vi "Read Controls.vi"(8 "error in (no error)":errorcluster, 11 "Test.Maui 2.0.Panels in":refnum<class "Test.Maui 2.0.Panels.lvclass">) -> (0 "error out":errorcluster, 2 "Controls":T1(array[cluster]), 3 "Test.Maui 2.0.Panels out":refnum<class "Test.Maui 2.0.Panels.lvclass">)   [LabVIEW 2020, in "Test.Maui 2.0.Panels.lvclass"]
uses:
  Test.Maui 2.0.Panels.lvclass
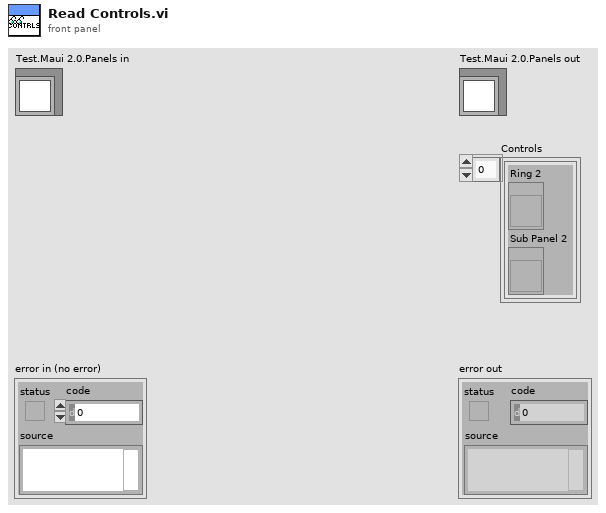
[diagram p1: front panel]
types:
  T1 = cluster{"Ring 2":refnum<vi>, "Sub Panel 2":refnum<vi>}[]
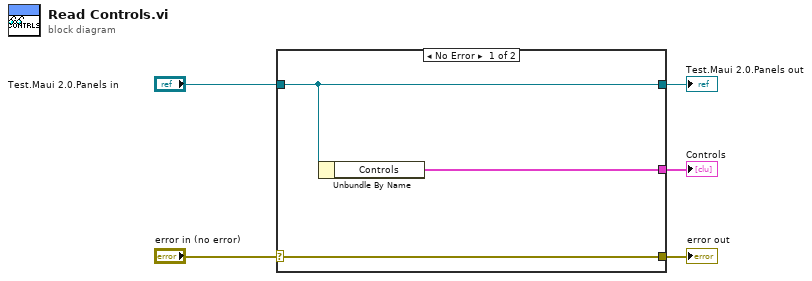
[diagram p0: block diagram]
diagram:
  n1 = case shown="No Error" "error in (no error)" {
    selector: "error in (no error)" -> [w8 w9]
    tunnel: [w8 w9] -> w4
    tunnel: [w7 w10] -> w2
    tunnel: "Test.Maui 2.0.Panels in" -> [w7 w10]
    tunnel: [w6 _] -> w1
    frame No Error {
      n2 = Unbundle By Name(w7) -> ("Controls"=w6:T1)
    }
    frame Error {
    }
  }
  "error out" <- w4
  "Test.Maui 2.0.Panels out" <- w2
  "Controls" <- w1
